vi "COMMAND_SetOrigin.vi"(8 "error in (no error)":errorcluster, 11 "StageDL090602SutterMP285 in":refnum<class "StageMMS2015ASI.lvclass">) -> (0 "error out":errorcluster, 3 "StageDL090602SutterMP285 out":refnum<class "StageMMS2015ASI.lvclass">)   [LabVIEW 2010, in "StageMMS2015ASI.lvclass"]
uses:
  StageMMS2015ASI.lvclass
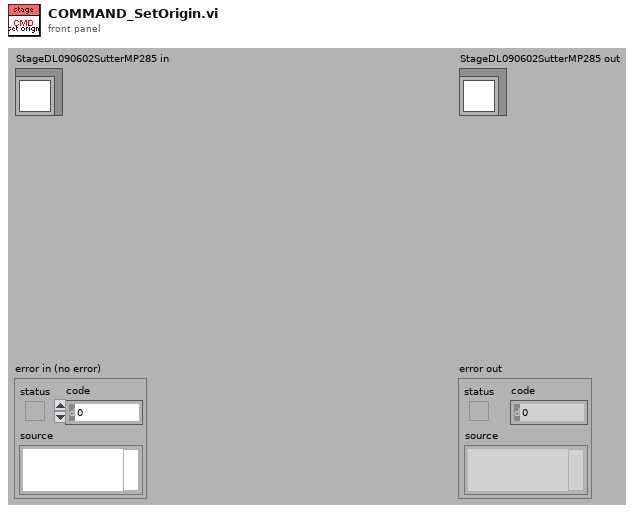
[diagram p1: front panel]
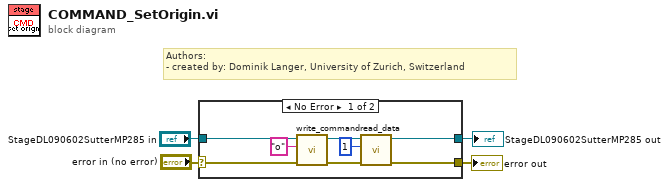
[diagram p0: block diagram]
diagram:
  # "Authors: \n- created by: Dominik Langer, University of Zurich, Switzerland"
  n1 = case shown="No Error" "error in (no error)" {
    selector: "error in (no error)" -> [w12 w14]
    tunnel: [w5 w14] -> w3
    tunnel: [w6 w13] -> w1
    tunnel: "StageDL090602SutterMP285 in" -> [w7 w13]
    frame No Error {
      n2 = call-dynamic "write_command.vi"("error in (no error)"=w12, "command (without terminating \"\\n\")"="o" ("command (without terminating \"\\n\")"), "DL090602SutterMP285Stage in"=w7) -> ("error out"=w10:errorcluster, "DL090602SutterMP285Stage out"=w9:refnum<class "StageMMS2015ASI.lvclass">)  [unwired: 7 in]
      n3 = call-dynamic "read_data.vi"("error in (no error)"=w10, "bytes to read"=u32 1, "DL090602SutterMP285Stage in"=w9) -> ("error out"=w5:errorcluster, "DL090602SutterMP285Stage out"=w6:refnum<class "StageMMS2015ASI.lvclass">)  [unwired: 6 in, 1 out]
    }
    frame Error {
    }
  }
  "error out" <- w3
  "StageDL090602SutterMP285 out" <- w1
